vi "Read Controllers.vi"   [LabVIEW 2014]
uses:
  Begin/Global RefNums.vi
  <vilib>/Rock Robotics/WPI/Joystick/WPI_JoystickGetSetRefNum.vi
  Begin/Global Variables.vi
types:
  T1 = typedef "WPI_JoystickDevRef.ctl" = cluster{"Device":T2}
  T2 = typedef "WPI_JoystickDeviceEnum.ctl" = enum16{"USB 0", "USB 1", "USB 2", "USB 3", "USB 4", "USB 5"}
  T3 = cluster{"Buttons[0]":bool, "Buttons[1]":bool, "Buttons[2]":bool, "Buttons[3]":bool, "Buttons[4]":bool, "Buttons[5]":bool, "Buttons[6]":bool, "Buttons[7]":bool, "Buttons[8]":bool}
  T4 = cluster{"Axes[0]":dbl, "Axes[1]":dbl, "Axes[2]":dbl, "Axes[3]":dbl, "Axes[4]":dbl, "Axes[5]":dbl, "Axes[6]":dbl, "Axes[7]":dbl, "Axes[8]":dbl}
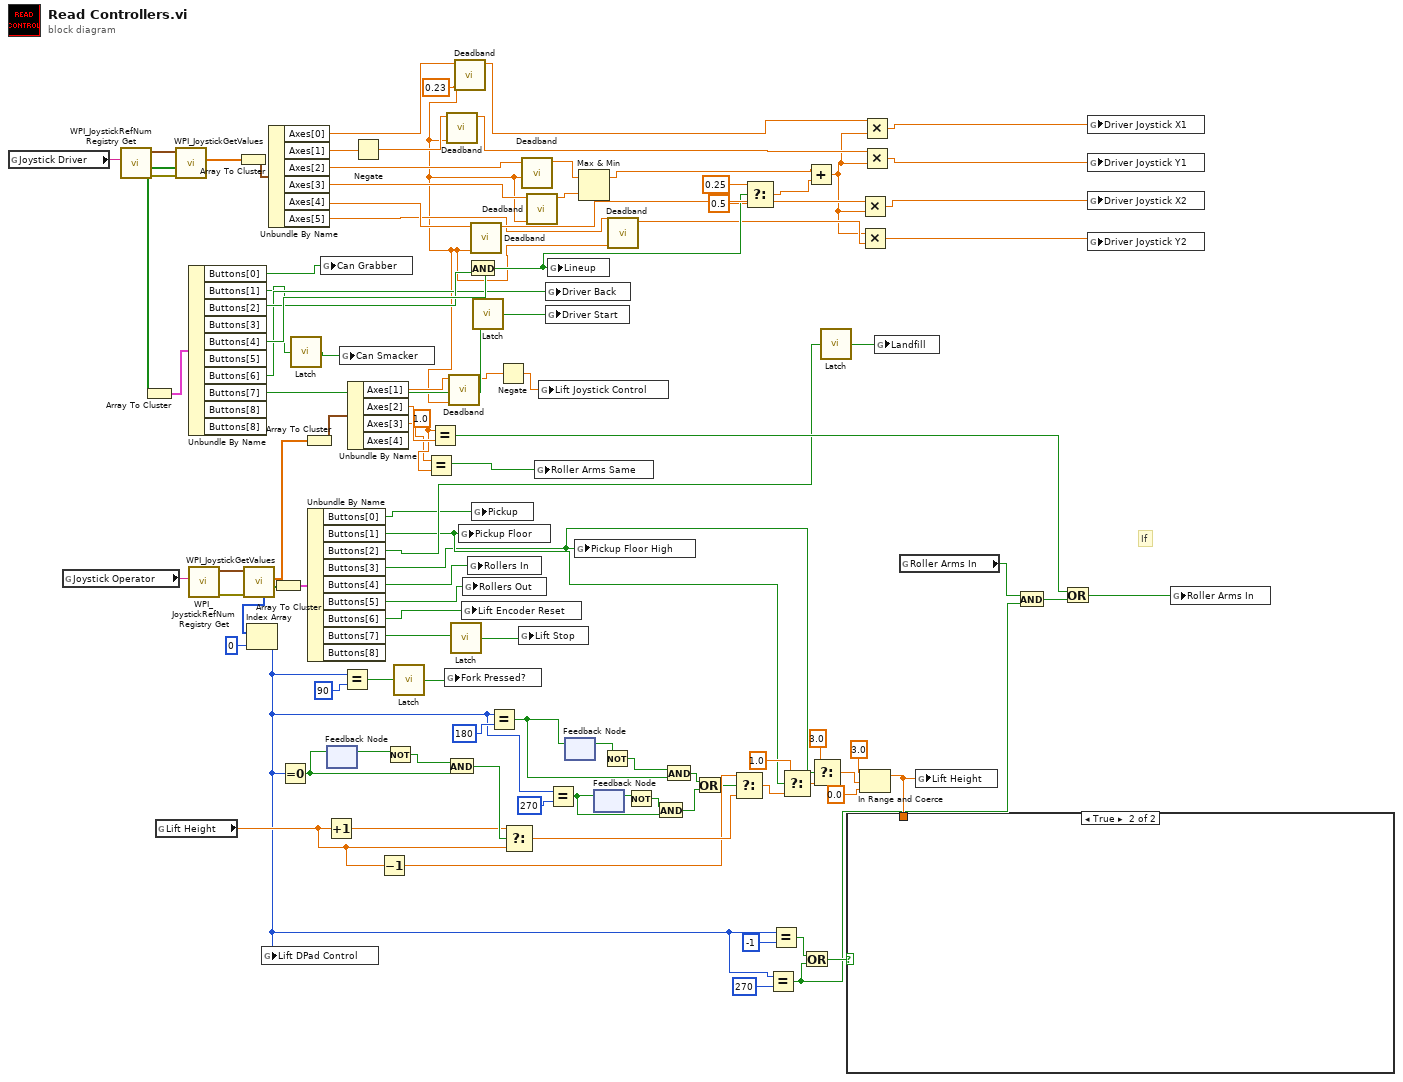
[diagram p0: block diagram]
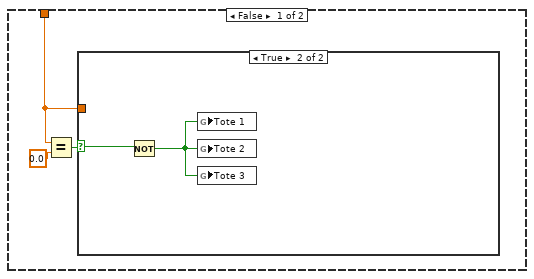
[diagram p2: hidden frame]
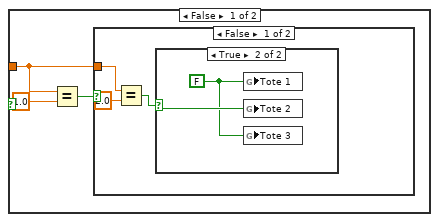
[diagram p3: hidden frame]
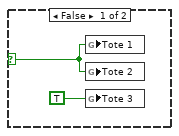
[diagram p4: hidden frame]
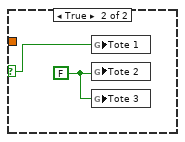
[diagram p5: hidden frame]
diagram:
  w48 = 1.0 ("x")
  w13 = 0.23 ("Value to Deadband (default of 0.1)")
  # "If"
  n1 = global read "Global RefNums.vi" "Joystick Driver"() -> (w105:string)
  n2 = global read "Global RefNums.vi" "Joystick Operator"() -> (w100:string)
  n3 = call <vilib>:"WPI_JoystickRefNum Registry Get.vi"("refnum name"=w105) -> ("error out"=w103:errorcluster, "JoystickDevRef"=w104:T1)  [unwired: 9 in]
  n4 = global read "Global Variables.vi" "Lift Height"() -> (w78:dbl)
  n5 = call <vilib>:"WPI_JoystickGetValues.vi"("error in (no error)"=w103, "JoystickDevRef"=w104) -> ("Buttons"=w97:bool[], "Axes"=w99:dbl[])  [unwired: 5 in, 3 out]
  n6 = Array To Cluster(array=w97) -> (cluster=w96:T3)
  n7 = Unbundle By Name(w96) -> ("Buttons[0]"=w31:bool, "Buttons[1]"=w8:bool, "Buttons[4]"=w46:bool, "Buttons[5]"=w45:bool, "Buttons[6]"=w15:bool, "Buttons[7]"=w74:bool)  [unwired: 4 out]
  n8 = call <vilib>:"WPI_JoystickRefNum Registry Get.vi"("refnum name"=w100) -> ("error out"=w102:errorcluster, "JoystickDevRef"=w101:T1)  [unwired: 9 in]
  n9 = Array To Cluster(array=w99) -> (cluster=w98:T4)
  n10 = call <vilib>:"WPI_JoystickGetValues.vi"("error in (no error)"=w102, "JoystickDevRef"=w101) -> ("Buttons"=w94:bool[], "Axes"=w71:dbl[], "POVs"=w90:i16[])  [unwired: 5 in, 2 out]
  n11 = Index Array(array=w90, index=0) -> (element=w38:i16)
  n12 = global write "Global Variables.vi" "Lift DPad Control"(w38) -> ()
  n13 = Unbundle By Name(w98) -> ("Axes[0]"=w95:dbl, "Axes[1]"=w58:dbl, "Axes[2]"=w30:dbl, "Axes[3]"=w29:dbl, "Axes[4]"=w59:dbl, "Axes[5]"=w14:dbl)
  n14 = Array To Cluster(array=w94) -> (cluster=w93:T3)
  n15 = Equal To 0?(x=w38) -> (x = 0?=w86:bool)
  n16 = call "Latch.vi"("Input"=w8) -> ("Output"=w9:bool)
  n17 = Array To Cluster(array=w71) -> (cluster=w70:T4)
  n18 = Unbundle By Name(w93) -> ("Buttons[0]"=w5:bool, "Buttons[1]"=w4:bool, "Buttons[2]"=w6:bool, "Buttons[3]"=w3:bool, "Buttons[4]"=w69:bool, "Buttons[5]"=w68:bool, "Buttons[6]"=w67:bool, "Buttons[7]"=w92:bool)  [unwired: 1 out]
  n19 = global write "Global Variables.vi" "Can Grabber"(w31) -> ()
  n20 = Increment(x=w78) -> (x+1=w84:dbl)
  n21 = feedback-in #1(w86) -> ()
  n22 = feedback #1() -> (w88:bool)  [unwired: 1 in]
  n23 = global write "Global Variables.vi" "Can Smacker"(w9) -> ()
  n24 = Equal?(x=w38, y=i16 90) -> (x = y?=w55:bool)
  n25 = Unbundle By Name(w70) -> ("Axes[1]"=w66:dbl, "Axes[2]"=w60:dbl, "Axes[3]"=w47:dbl)  [unwired: 1 out]
  n26 = Negate(x=w58) -> (-x=w57:dbl)
  n27 = Decrement(x=w78) -> (x-1=w77:dbl)
  n28 = Not(x=w88) -> (.not. x?=w87:bool)
  n29 = call "Latch.vi"("Input"=w55) -> ("Output"=w54:bool)
  n30 = Equal?(x=w47, y=w48) -> (x = y?=w2:bool)
  n31 = Equal?(x=w48, y=w60) -> (x = y?=w50:bool)
  n32 = global write "Global Variables.vi" "Fork Pressed?"(w54) -> ()
  n33 = call "Deadband.vi"("Value to Deadband (default of 0.1)"=w13, "Value"=w57) -> ("Deadbanded Value"=w24:dbl)  [unwired: 9 in]
  n34 = And(x=w87, y=w86) -> (x .and. y?=w85:bool)
  n35 = call "Deadband.vi"("Value to Deadband (default of 0.1)"=w13, "Value"=w66) -> ("Deadbanded Value"=w64:dbl)  [unwired: 9 in]
  n36 = call "Latch.vi"("Input"=w92) -> ("Output"=w91:bool)
  n37 = call "Deadband.vi"("Value to Deadband (default of 0.1)"=w13, "Value"=w95) -> ("Deadbanded Value"=w25:dbl)  [unwired: 9 in]
  n38 = global write "Global Variables.vi" "Pickup Floor"(w4) -> ()
  n39 = global write "Global Variables.vi" "Lift Encoder Reset"(w67) -> ()
  n40 = global write "Global Variables.vi" "Rollers Out"(w68) -> ()
  n41 = And(x=w46, y=w45) -> (x .and. y?=w20:bool)
  n42 = global write "Global Variables.vi" "Rollers In"(w69) -> ()
  n43 = call "Deadband.vi"("Value to Deadband (default of 0.1)"=w13, "Value"=w59) -> ("Deadbanded Value"=w23:dbl)  [unwired: 9 in]
  n44 = global write "Global Variables.vi" "Pickup"(w5) -> ()
  n45 = call "Latch.vi"("Input"=w74) -> ("Output"=w73:bool)
  n46 = Equal?(x=w38, y=i16 180) -> (x = y?=w82:bool)
  n47 = Negate(x=w64) -> (-x=w63:dbl)
  n48 = Select(t=w84, s=w85, f=w78) -> (s? t:f=w79:dbl)
  n49 = global write "Global Variables.vi" "Lift Stop"(w91) -> ()
  n50 = call "Deadband.vi"("Value to Deadband (default of 0.1)"=w13, "Value"=w30) -> ("Deadbanded Value"=w27:dbl)  [unwired: 9 in]
  n51 = call "Deadband.vi"("Value to Deadband (default of 0.1)"=w13, "Value"=w29) -> ("Deadbanded Value"=w28:dbl)  [unwired: 9 in]
  n52 = global write "Global Variables.vi" "Roller Arms Same"(w2) -> ()
  n53 = global write "Global Variables.vi" "Lift Joystick Control"(w63) -> ()
  n54 = global write "Global Variables.vi" "Driver Back"(w15) -> ()
  n55 = global write "Global Variables.vi" "Driver Start"(w73) -> ()
  n56 = global write "Global Variables.vi" "Lineup"(w20) -> ()
  n57 = Equal?(x=w38, y=i16 270) -> (x = y?=w44:bool)
  n58 = feedback #2() -> (w81:bool)  [unwired: 1 in]
  n59 = feedback-in #2(w82) -> ()
  n60 = global write "Global Variables.vi" "Pickup Floor High"(w3) -> ()
  n61 = Max & Min(x=w27, y=w28) -> (max(x,y)=w26:dbl)  [unwired: 1 out]
  n62 = feedback #3() -> (w42:bool)  [unwired: 1 in]
  n63 = feedback-in #3(w44) -> ()
  n64 = Not(x=w81) -> (.not. x?=w80:bool)
  n65 = call "Deadband.vi"("Value to Deadband (default of 0.1)"=w13, "Value"=w14) -> ("Deadbanded Value"=w12:dbl)  [unwired: 9 in]
  n66 = Not(x=w42) -> (.not. x?=w43:bool)
  n67 = And(x=w43, y=w44) -> (x .and. y?=w40:bool)
  n68 = And(x=w80, y=w82) -> (x .and. y?=w41:bool)
  n69 = Or(x=w41, y=w40) -> (x .or. y?=w39:bool)
  n70 = Select(t=w77, s=w39, f=w79) -> (s? t:f=w36:dbl)
  n71 = Select(t=0.25, s=w20, f=0.5) -> (s? t:f=w18:dbl)
  n72 = Equal?(x=w38, y=i16 270) -> (x = y?=w51:bool)
  n73 = Equal?(x=w38, y=i16 -1) -> (x = y?=w62:bool)
  n74 = Select(t=1.0, s=w4, f=w36) -> (s? t:f=w34:dbl)
  n75 = Or(x=w62, y=w51) -> (x .or. y?=w53:bool)
  n76 = Add(x=w26, y=w18) -> (x+y=w11:dbl)
  n77 = Select(t=3.0, s=w3, f=w34) -> (s? t:f=w32:dbl)
  n78 = call "Latch.vi"("Input"=w6) -> ("Output"=w7:bool)
  n79 = Multiply(x=w23, y=w11) -> (x*y=w22:dbl)
  n80 = Multiply(x=w11, y=w12) -> (x*y=w10:dbl)
  n81 = In Range and Coerce(upper limit=3.0, x=w32, lower limit=0.0) -> (coerced(x)=w72:dbl)  [unwired: 1 out]
  n82 = case shown="True" w53 {
    tunnel: w72 -> [w108 _]
    frame False {
      n83 = Equal?(x=w108, y=0.0) -> (x = y?=w107:bool)
      n84 = case shown="True" w107 {
        selector: w107 -> [_ w122]
        tunnel: w108 -> [w109 _]
        frame False {
          n85 = Equal?(x=w109, y=1.0) -> (x = y?=w110:bool)
          n86 = case shown="False" w110 {
            selector: w110 -> [_ w119]
            tunnel: w109 -> [w114 _]
            frame False {
              n87 = Equal?(x=w114, y=2.0) -> (x = y?=w112:bool)
              n88 = case shown="True" w112 {
                selector: w112 -> [w115 w118]
                frame False {
                  n89 = global write "Global Variables.vi" "Tote 1"(w115) -> ()
                  n90 = global write "Global Variables.vi" "Tote 2"(w115) -> ()
                  n91 = global write "Global Variables.vi" "Tote 3"(TRUE ("Tote 2")) -> ()
                }
                frame True {
                  w117 = FALSE ("Tote 0")
                  n92 = global write "Global Variables.vi" "Tote 1"(w117) -> ()
                  n93 = global write "Global Variables.vi" "Tote 2"(w118) -> ()
                  n94 = global write "Global Variables.vi" "Tote 3"(w117) -> ()
                }
              }
            }
            frame True {
              w120 = FALSE ("Tote 1")
              n95 = global write "Global Variables.vi" "Tote 1"(w119) -> ()
              n96 = global write "Global Variables.vi" "Tote 2"(w120) -> ()
              n97 = global write "Global Variables.vi" "Tote 3"(w120) -> ()
            }
          }
        }
        frame True {
          n98 = Not(x=w122) -> (.not. x?=w121:bool)
          n99 = global write "Global Variables.vi" "Tote 1"(w121) -> ()
          n100 = global write "Global Variables.vi" "Tote 2"(w121) -> ()
          n101 = global write "Global Variables.vi" "Tote 3"(w121) -> ()
        }
      }
    }
    frame True {
    }
  }
  n102 = Multiply(x=w25, y=w11) -> (x*y=w16:dbl)
  n103 = Multiply(x=w24, y=w11) -> (x*y=w21:dbl)
  n104 = global write "Global Variables.vi" "Landfill"(w7) -> ()
  n105 = global read "Global Variables.vi" "Roller Arms In"() -> (w52:bool)
  n106 = global write "Global Variables.vi" "Lift Height"(w72) -> ()
  n107 = And(x=w52, y=w51) -> (x .and. y?=w49:bool)
  n108 = Or(x=w50, y=w49) -> (x .or. y?=w1:bool)
  n109 = global write "Global Variables.vi" "Driver Joystick X1"(w16) -> ()
  n110 = global write "Global Variables.vi" "Driver Joystick Y1"(w21) -> ()
  n111 = global write "Global Variables.vi" "Driver Joystick X2"(w22) -> ()
  n112 = global write "Global Variables.vi" "Driver Joystick Y2"(w10) -> ()
  n113 = global write "Global Variables.vi" "Roller Arms In"(w1) -> ()
